vi "ORS_PathAddExtension.vi"(7 "new extension":string="dat", 11 "path":path=path "c:/test") -> (3 "appended path":path=path "c:/test.dat")   [LabVIEW 2024]
doc: "Adds new file extension.New extension has to be without leading dot. Old extension, if any, will become part of new file name."
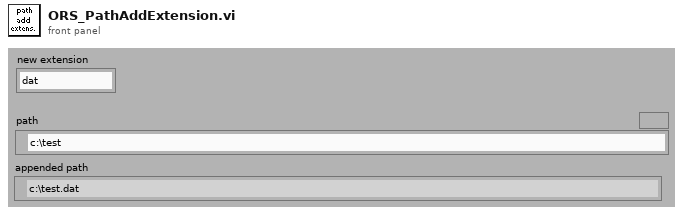
[diagram p1: front panel]
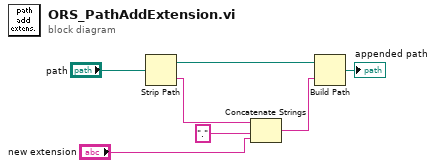
[diagram p0: block diagram]
diagram:
  n1 = Strip Path(path="path") -> (stripped path=w6:path, name=w2:string)
  n2 = Concatenate Strings(w2, ".", "new extension") -> (w7:string)
  n3 = Build Path(base path=w6, name or relative path=w7) -> (appended path=→"appended path":path)
